vi "Send_UIReadCtrl.vi"(6 "HighPriority (F)":bool, 8 "error in":errorcluster, 10 "Control Label":string, 11 "Queue in":refnum<queue>) -> (0 "error out":errorcluster, 1 "Control Data":variant, 2 "Found":bool, 3 "Ctl_Refnum":refnum<vi>, 4 "ReadError":bool)   [LabVIEW 2018, in "UI_Library.lvlib"]
uses:
  UI_Library.lvlib
panel:
  in  "Timeout_ms (500)":i32=500
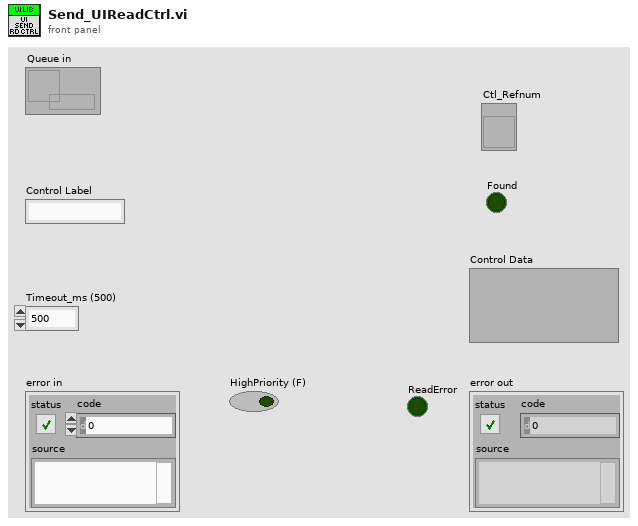
[diagram p1: front panel]
types:
  T1 = cluster{"Ctl_Refnum":refnum<vi>, "Found":bool, "Control Data":variant, "error out":errorcluster}
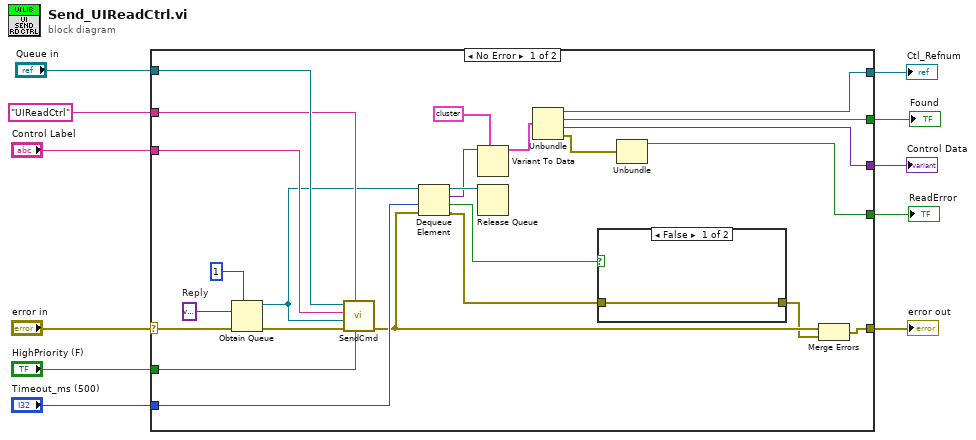
[diagram p0: block diagram]
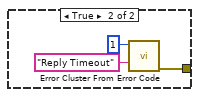
[diagram p2: hidden frame]
diagram:
  n1 = case shown="No Error" "error in" {
    selector: "error in" -> [w32 w40]
    tunnel: "Queue in" -> [w35 _]
    tunnel: "Control Label" -> [w28 _]
    tunnel: "UIReadCtrl" ("UICmd") -> [w29 _]
    tunnel: "HighPriority (F)" -> [w34 _]
    tunnel: [w17 w40] -> w11
    tunnel: "Timeout_ms (500)" -> [w25 _]
    tunnel: [w21 _] -> w4
    tunnel: [w20 _] -> w3
    tunnel: [w19 _] -> w2
    tunnel: [w12 _] -> w1
    frame No Error {
      w33 = variant  # Reply
      n2 = Obtain Queue(max queue size (-1, unlimited)=1, element data type=w33, error in (no error)=w32) -> (queue out=w27:refnum<queue>, error out=w30:errorcluster)  [unwired: 2 in, 1 out]
      n3 = call "SendCmd.vi"("HighPriority (F)"=w34, "UICmd"=w29, "error in"=w30, "Control Data"=w27, "Control Label"=w28, "Queue in"=w35) -> ("error out"=w23:errorcluster)  [unwired: 5 in]
      n4 = Dequeue Element(queue=w27, timeout in ms (-1)=w25, error in (no error)=w23) -> (queue out=w31:refnum<queue>, element=w24:variant, timed out?=w18:bool, error out=w15:errorcluster)
      n5 = Variant To Data(type=T1 {"Ctl_Refnum"=refnum, "Found"=FALSE, "Control Data"=variant, "error out"={"status"=FALSE, "code"=0, "source"=""}}, Variant=w24) -> (data=w22:T1)  [unwired: 1 in, 1 out]
      n6 = Release Queue(queue=w31) -> ()  [unwired: 2 in, 3 out]
      n7 = Unbundle(w22) -> ("Ctl_Refnum"=w21:refnum<vi>, "Found"=w20:bool, "Control Data"=w19:variant, "error out"=w13:errorcluster)
      n8 = case shown="False" w18 {
        tunnel: [w36 w38] -> w16
        tunnel: w15 -> [w36 _]
        frame False {
        }
        frame True {
          n9 = call <vilib>:"Error Cluster From Error Code.vi"("error message (\"\")"="Reply Timeout" ("error message (\"\")"), "error code (0)"=1) -> ("error out"=w38:errorcluster)  [unwired: 7 in]
        }
      }
      n10 = Unbundle(w13) -> ("status"=w12:bool)  [unwired: 2 out]
      n11 = Merge Errors(w23, w16) -> (w17:errorcluster)
    }
    frame Error {
    }
  }
  "error out" <- w11
  "Ctl_Refnum" <- w4
  "Control Data" <- w2
  "Found" <- w3
  "ReadError" <- w1
